vi "cm-pixel(SubVI).vi"(11 "NavData Out in":T1) -> (3 "1 pixel equals to: (in cm)":dbl format="%.2f")   [LabVIEW 2014]
uses:
  <vilib>/LVH/AR Drone Toolkit/Decode NavData/Typedefs/NavData Demo.ctl
  <vilib>/LVH/AR Drone Toolkit/AR Drone.lvlib
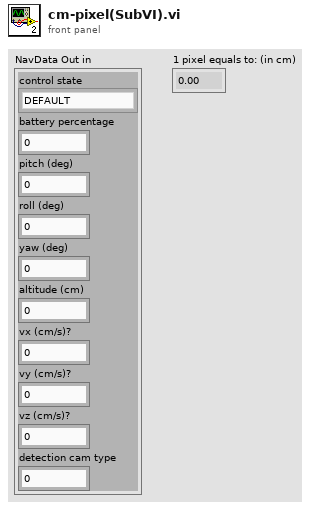
[diagram p1: front panel]
types:
  T1 = typedef "AR Drone.lvlib/NavData Demo.ctl" = cluster{"control state":enum32{"DEFAULT", "INIT", "LANDING", "FLYING", "HOVERING", "TEST", "TRANS_TAKEOFF", "TRANS_GOTOFIX", "TRANS_LANDING"}, "battery percentage":u32, "pitch (deg)":sgl, "roll (deg)":sgl, "yaw (deg)":sgl, "altitude (cm)":u32, "vx (cm/s)?":sgl, "vy (cm/s)?":sgl, "vz (cm/s)?":sgl, "detection cam type":u32}
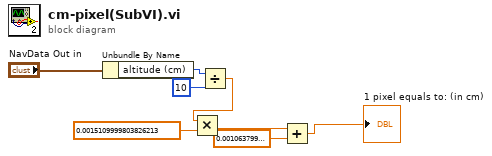
[diagram p0: block diagram]
diagram:
  n1 = Unbundle By Name("NavData Out in") -> ("altitude (cm)"=w3:u32)
  n2 = Divide(x=w3, y=u32 10) -> (x/y=w1:dbl)
  n3 = Multiply(x=w1, y=sgl 0.001511) -> (x*y=w7:dbl)
  n4 = Add(x=w7, y=sgl 0.0010638) -> (x+y=→"1 pixel equals to: (in cm)":dbl)
